vi "CRYExchange Symbol String.vi"(8 "nData":i32, 9 "sData":string, 11 "sAction":string) -> (2 "nData out":i32=81, 3 "sData out":string)   [LabVIEW 2013]
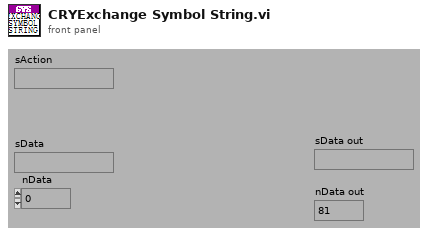
[diagram p1: front panel]
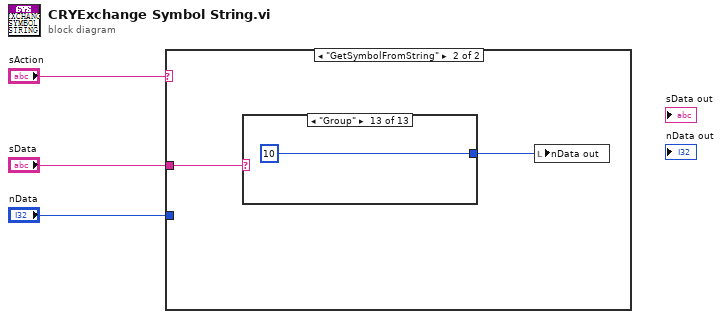
[diagram p0: block diagram]
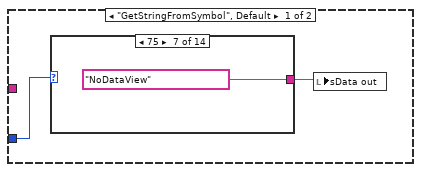
[diagram p2: hidden frame]
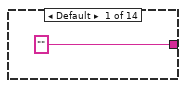
[diagram p3: hidden frame]
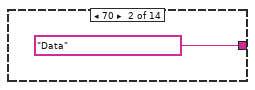
[diagram p4: hidden frame]
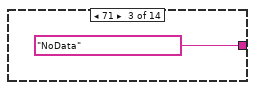
[diagram p5: hidden frame]
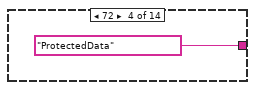
[diagram p6: hidden frame]
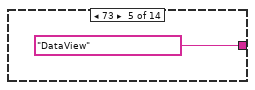
[diagram p7: hidden frame]
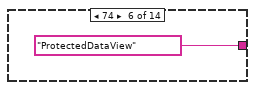
[diagram p8: hidden frame]
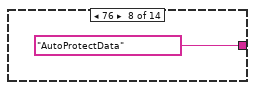
[diagram p9: hidden frame]
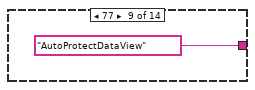
[diagram p10: hidden frame]
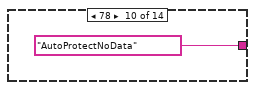
[diagram p11: hidden frame]
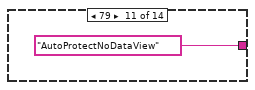
[diagram p12: hidden frame]
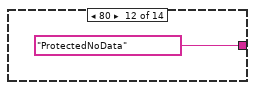
[diagram p13: hidden frame]
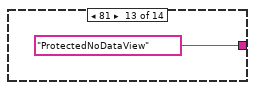
[diagram p14: hidden frame]
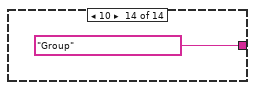
[diagram p15: hidden frame]
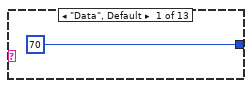
[diagram p16: hidden frame]
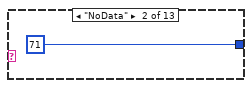
[diagram p17: hidden frame]
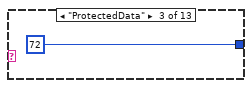
[diagram p18: hidden frame]
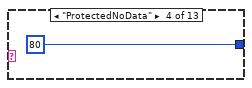
[diagram p19: hidden frame]
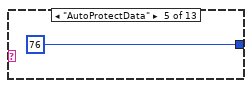
[diagram p20: hidden frame]
diagram:
  n1 = case shown="\"GetSymbolFromString\"" "sAction" {
    tunnel: "sData" -> [_ w21]
    tunnel: "nData" -> [w5 _]
    frame "GetStringFromSymbol", Default {
      n2 = case shown="75" w5 {
        tunnel: ["" ("name or relative path") "Data" ("name or relative path") "NoData" ("name or relative path") "ProtectedData" ("name or relative path") "DataView" ("name or relative path") "ProtectedDataView" ("name or relative path") "NoDataView" ("name or relative path") "AutoProtectData" ("name or relative path") "AutoProtectDataView" ("name or relative path") "AutoProtectNoData" ("name or relative path") "AutoProtectNoDataView" ("name or relative path") "ProtectedNoData" ("name or relative path") "ProtectedNoDataView" ("name or relative path") "Group" ("name or relative path")] -> w4
        frame Default {
        }
        frame 70 {
        }
        frame 71 {
        }
        frame 72 {
        }
        frame 73 {
        }
        frame 74 {
        }
        frame 75 {
        }
        frame 76 {
        }
        frame 77 {
        }
        frame 78 {
        }
        frame 79 {
        }
        frame 80 {
        }
        frame 81 {
        }
        frame 10 {
        }
      }
      n3 = local write "sData out"(w4) -> ()
    }
    frame "GetSymbolFromString" {
      n4 = case shown="\"Group\"" w21 {
        tunnel: [70 ("index") 71 ("index") 72 ("index") 80 ("index") 76 ("index") 78 ("index") 73 ("index") 75 ("index") 77 ("index") 79 ("index") 74 ("index") 81 ("index") 10 ("index")] -> w20
        frame "Data", Default {
        }
        frame "NoData" {
        }
        frame "ProtectedData" {
        }
        frame "ProtectedNoData" {
        }
        frame "AutoProtectData" {
        }
        frame "AutoProtectNoData" {
        }
        frame "DataView" {
        }
        frame "NoDataView" {
        }
        frame "AutoProtectDataView" {
        }
        frame "AutoProtectNoDataView" {
        }
        frame "ProtectedDataView" {
        }
        frame "ProtectedNoDataView" {
        }
        frame "Group" {
        }
      }
      n5 = local write "nData out"(w20) -> ()
    }
  }
